vi "Write and Get Channel Readings.vi"(8 "error in":errorcluster, 9 "Readings":waveform(dbl)[](array[waveform]), 10 "Channel":string, 11 "BufferLossless in":refnum<class "Buffer Lossless Base.lvclass">=refnum) -> (0 "error out":errorcluster, 2 "Reading":waveform(dbl), 3 "BufferLossless out":refnum<class "Buffer Lossless Base.lvclass">)   [LabVIEW 2024, in "Buffer Lossless.lvclass"]
uses:
  Buffer Lossless.lvclass
  Buffer Lossless.lvclass/Buffer Lossless.ctl
  Buffer Lossless Base.lvclass
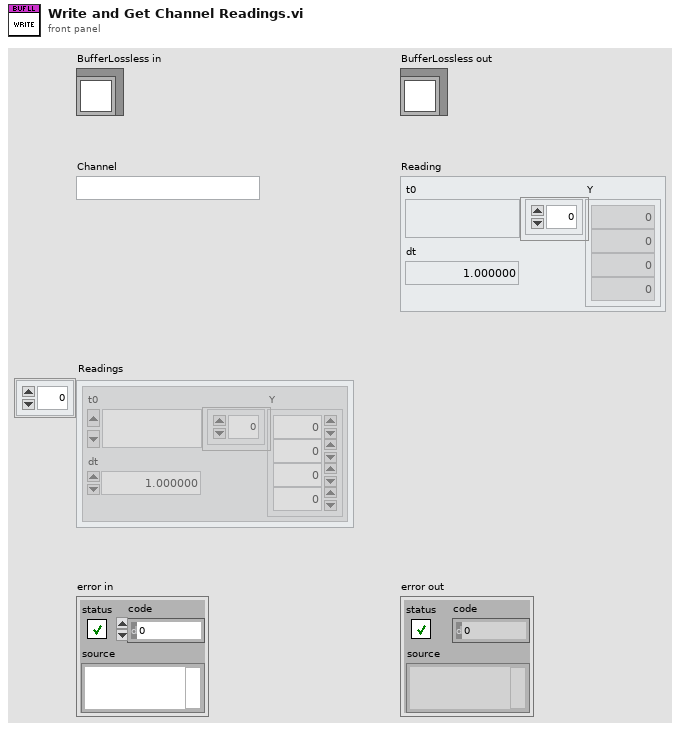
[diagram p1: front panel]
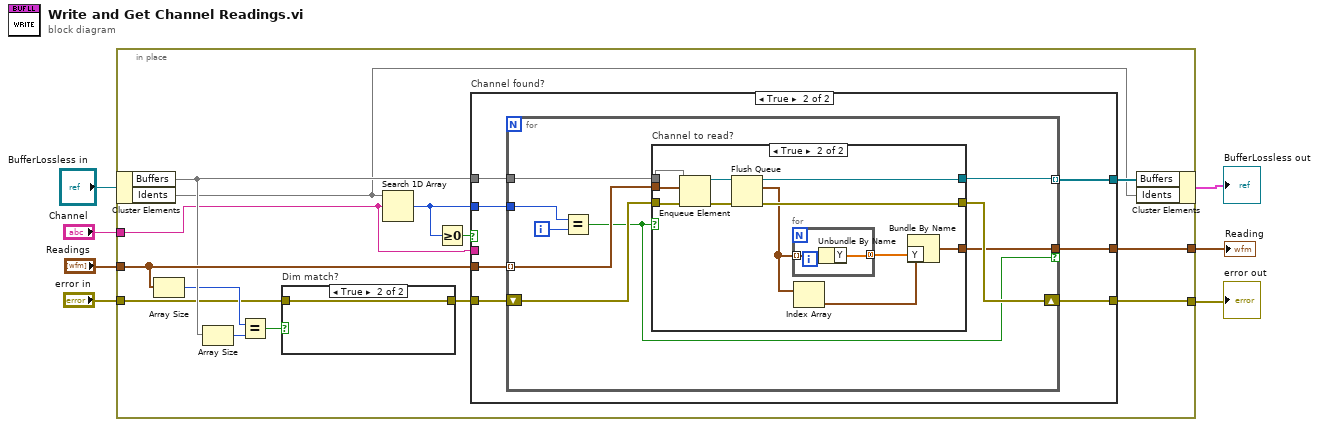
[diagram p0: block diagram]
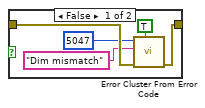
[diagram p2: hidden frame]
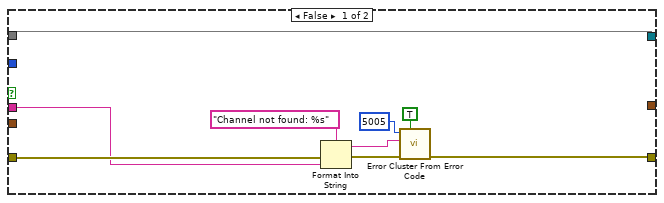
[diagram p3: hidden frame]
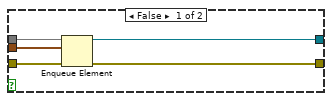
[diagram p4: hidden frame]
diagram:
  n1 = in-place {
    in-place-border: "Readings" -> [w18]
    in-place-border: "error in" -> [w13]
    in-place-border: [w21] -> w2
    in-place-border: "Channel" -> [w8]
    in-place-border: [w9] -> w1
    n2 = in-place-cluster #1("BufferLossless in") -> ("Buffers"=w17, "Idents"=w10)
    n3 = Array Size(array=w18) -> (size(s)=w14:i32)
    n4 = Array Size(array=w17) -> (size(s)=w15:i32)
    n5 = Equal?(x=w14, y=w15) -> (x = y?=w16:bool)
    n6 = case "Dim match?" shown="True" w16 {
      tunnel: w13 -> [w26 w27]
      tunnel: [w25 w27] -> w12
      frame False {
        n7 = call <vilib>:"Error Cluster From Error Code.vi"("show call chain? (False)"=TRUE, "error in (no error)"=w26, "error message (\"\")"="Dim mismatch" ("error message (\"\")"), "error code (0)"=5047) -> ("error out"=w25:errorcluster)  [unwired: 5 in]
      }
      frame True {
      }
    }
    n8 = Search 1D Array(1D array=w10, element=w8) -> (index of element=w20:i32)  [unwired: 1 in]
    n9 = Greater Or Equal To 0?(x=w20) -> (x >= 0?=w19:bool)
    n10 = case "Channel found?" shown="True" w19 {
      tunnel: w12 -> [w31 w43]
      tunnel: [w30 w42] -> w21
      tunnel: w17 -> [w29 w39]
      tunnel: w20 -> [_ w41]
      tunnel: w18 -> [_ w40]
      tunnel: [w29 w38] -> w11
      tunnel: [_ w37] -> w9
      tunnel: w8 -> [w28 _]
      frame False {
        n11 = Format Into String(format string="Channel not found: %s", error in=w31, w28) -> (resulting string=w32:string, error out=w34:errorcluster)  [unwired: 1 in]
        n12 = call <vilib>:"Error Cluster From Error Code.vi"("show call chain? (False)"=TRUE, "error in (no error)"=w34, "error message (\"\")"=w32, "error code (0)"=5005) -> ("error out"=w30:errorcluster)  [unwired: 5 in]
      }
      frame True {
        n13 = for {
          tunnel: w41 -> [w48]
          shift-right: [w49] -> w42
          shift-left: w43 -> [w50]
          tunnel: w40 -> [w51] mode=indexing
          tunnel: w39 -> [w52]
          tunnel: [w46] -> w38 mode=indexing
          tunnel: [w45] -> w37 if=w44
          i -> [w47]
          n14 = Equal?(x=w48, y=w47) -> (x = y?=w44:bool)
          n15 = case "Channel to read?" shown="True" w44 {
            tunnel: w52 -> [w57 w61]
            tunnel: w51 -> [w56 w59]
            tunnel: w50 -> [w55 w67]
            tunnel: [w54 w64] -> w49
            tunnel: [w53 w68] -> w46
            tunnel: [_ w63] -> w45
            frame False {
              n16 = Enqueue Element(queue=w57, element=w56, error in (no error)=w55) -> (queue out=w53:refnum<queue>, error out=w54:errorcluster)  [unwired: 1 in, 1 out]
            }
            frame True {
              n17 = Enqueue Element(queue=w61, element=w59, error in (no error)=w67) -> (queue out=w60:refnum<queue>, error out=w62:errorcluster)  [unwired: 1 in, 1 out]
              n18 = Flush Queue(queue=w60, error in (no error)=w62) -> (queue out=w68:refnum<queue>, remaining elements=w58:waveform(dbl)[], error out=w64:errorcluster)
              n19 = for {
                tunnel: w58 -> [w70] mode=indexing
                tunnel: [w69] -> w65 mode=concatenating
                n20 = Unbundle By Name(w70) -> ("Y"=w69:dbl[])
              }
              n21 = Index Array(array=w58) -> (element=w66:waveform(dbl))  [unwired: 1 in]
              n22 = Bundle By Name(cluster=w66, "Y"=w65) -> (w63:waveform(dbl))
            }
          }
        }
      }
    }
    n23 = in-place-cluster #1("Buffers"=w11, "Idents"=w10) -> (→"BufferLossless out":cluster{})
  }
  "error out" <- w2
  "Reading" <- w1
